vi "brace_space_inside_brace.vi"(8 "error in (no error)":errorcluster, 11 "Instrument Command In":string="TRIGger:AND:ENABle {{ON | 1} | {OFF | 0}} ") -> (0 "error out":errorcluster, 2 "Boolean":bool, 3 "Instrument Command Out":string)   [LabVIEW 2018]
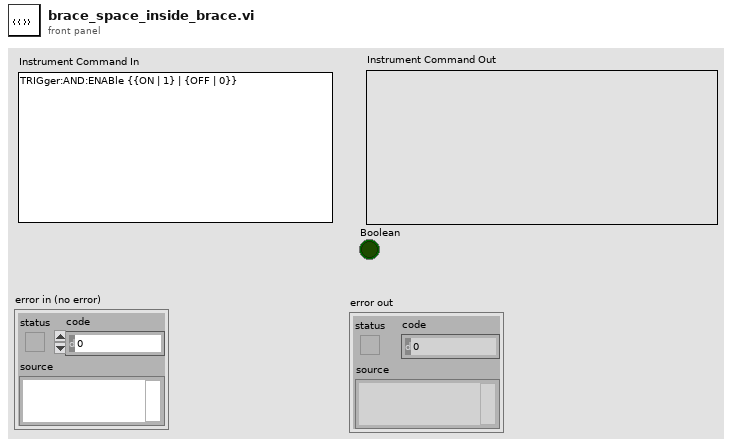
[diagram p1: front panel]
types:
  T1 = cluster{"Start Sting":string, "End String":string}[]
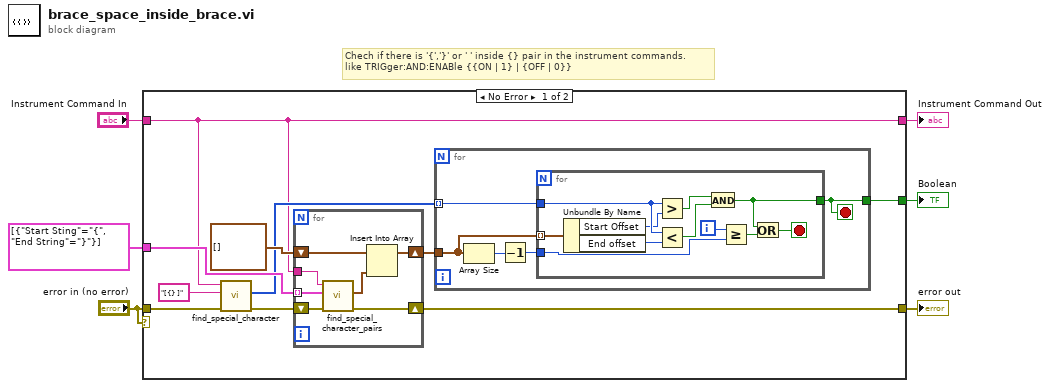
[diagram p0: block diagram]
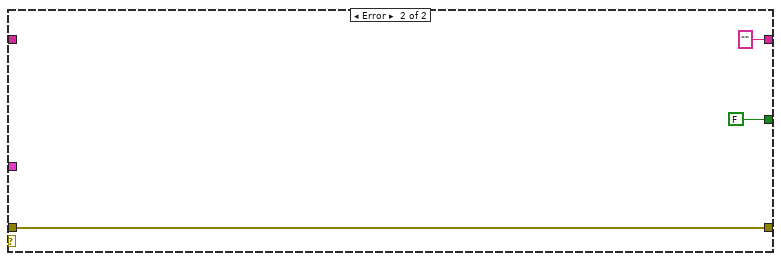
[diagram p2: hidden frame]
diagram:
  # "Chech if there is '{','}' or ' ' inside {} pair in the instrument commands. \nlike TRIGger:AND:ENABle {{ON | 1} | {OFF | 0}}"
  n1 = case shown="No Error" "error in (no error)" {
    tunnel: [w8 "" ("result string")] -> w6
    tunnel: "Instrument Command In" -> [w8 _]
    tunnel: "error in (no error)" -> [w16 w41]
    tunnel: [w10 w41] -> w3
    tunnel: T1 [{"Start Sting"="{", "End String"="}"}] -> [w14 _]
    tunnel: [w9 FALSE] -> w1
    frame No Error {
      n2 = call "find_special_character.vi"("error in (no error)"=w16, "Character"="[{} ]", "Command String"=w8) -> ("error out"=w13:errorcluster, "Offset Array"=w11:i32[])  [unwired: 7 out]
      n3 = for {
        tunnel: w8 -> [w39]
        tunnel: w14 -> [w38] mode=indexing
        shift-right: [w35] -> w7
        shift-left: cluster{"Start Offset":i32, "End offset":i32}[] [] ("Pair Offset") -> [w36]
        shift-right: [w33] -> w10
        shift-left: w13 -> [w34]
        n4 = call "find_special_character_pairs.vi"("error in (no error)"=w34, "String Pair"=w38, "Command String"=w39) -> ("error out"=w33:errorcluster, "Pair Offset"=w37:cluster{"Start Offset":i32, "End offset":i32}[])  [unwired: 7 out]
        n5 = Insert Into Array(array=w36, new element=w37) -> (w35:cluster{"Start Offset":i32, "End offset":i32}[])  [unwired: 1 in]
      }
      n6 = for {
        tunnel: w11 -> [w21] mode=indexing
        tunnel: [w17] -> w9
        tunnel: w7 -> [w18]
        stop <- w17 stop-if-true
        n7 = Array Size(array=w18) -> (size(s)=w20:i32)
        n8 = Decrement(x=w20) -> (x-1=w19:i32)
        n9 = for {
          tunnel: w21 -> [w30]
          tunnel: w19 -> [w28]
          tunnel: [w25] -> w17
          tunnel: w18 -> [w24] mode=indexing
          i -> [w29]
          stop <- w26 stop-if-true
          n10 = Unbundle By Name(w24) -> ("Start Offset"=w22:i32, "End offset"=w23:i32)
          n11 = Greater?(x=w30, y=w22) -> (0:w32:bool)
          n12 = Less?(x=w30, y=w23) -> (x < y?=w31:bool)
          n13 = And(x=w32, y=w31) -> (x .and. y?=w25:bool)
          n14 = Greater Or Equal?(x=w29, y=w28) -> (x >= y?=w27:bool)
          n15 = Or(x=w25, y=w27) -> (x .or. y?=w26:bool)
        }
      }
    }
    frame Error {
    }
  }
  "Instrument Command Out" <- w6
  "error out" <- w3
  "Boolean" <- w1
